vi "FolderMon stop.vi"(4 "error in (no error)":errorcluster) -> (0 "error out":errorcluster)   [LabVIEW 2011]
uses:
  FolderMon events.ctl
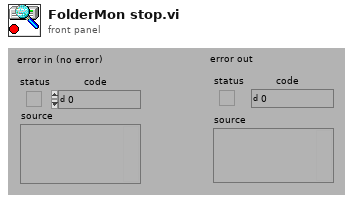
[diagram p1: front panel]
types:
  T1 = typedef "FolderMon events.ctl" = enum16{"stop", "update"}
  T2 = enum32{"Bad", "Idle", "Run top level", "Running"}
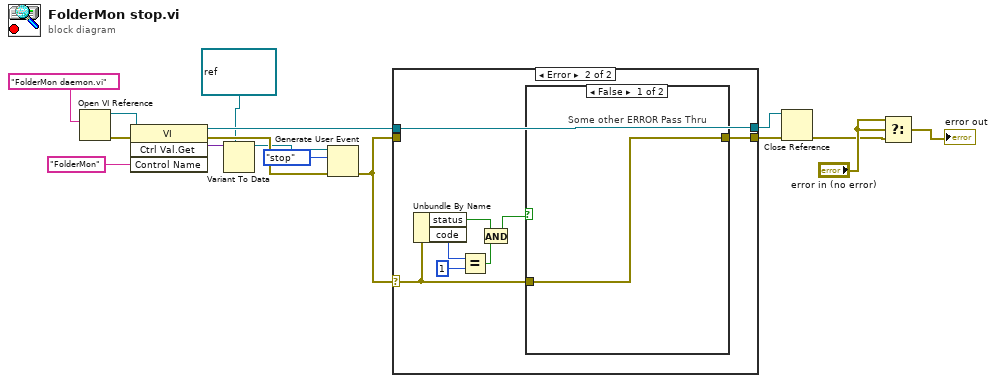
[diagram p0: block diagram]
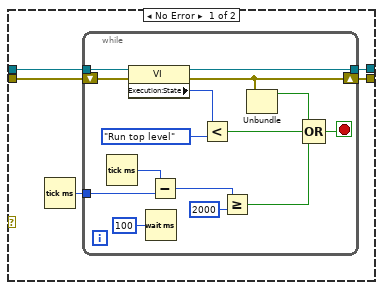
[diagram p2: hidden frame]
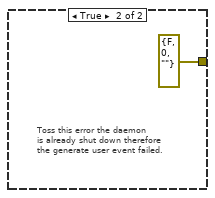
[diagram p3: hidden frame]
diagram:
  w3 = refnum<user-event> refnum items=["stop", "update"] ("FolderMon")
  n1 = Open VI Reference(vi path="FolderMon daemon.vi") -> (vi reference=w15:refnum<vi>, error out=w14:errorcluster)  [unwired: 1 in, 4 out]
  n2 = invoke class="VI" method="Ctrl Val.Get"(reference=w15, error in=w14, "Control Name"="FolderMon") -> (reference out=w12:refnum<vi>, error out=w9:errorcluster, "Get Control Value Variant"=w2:variant)  [unwired: 1 in, 1 out]
  n3 = Variant To Data(type=w3, Variant=w2) -> (data=w1:refnum<user-event>)  [unwired: 1 in, 1 out]
  n4 = Generate User Event(user event=w1, event data cluster=FolderMon_events."stop" ("event data"), error in=w9) -> (error out=w7:errorcluster)  [unwired: 1 out]
  n5 = case shown="Error" w7 {
    selector: w7 -> [_ w38]
    tunnel: w12 -> [w21 w37]
    tunnel: [w19 w39] -> w11
    tunnel: [w18 w37] -> w10
    tunnel: w7 -> [w17 _]
    frame No Error {
      n6 = Tick Count (ms)() -> (millisecond timer value=w20:u32)
      n7 = while {
        shift-right: [w27] -> w19
        shift-left: w17 -> [w33]
        tunnel: w21 -> [w34]
        tunnel: w20 -> [w31]
        tunnel: [w22] -> w18
        stop <- w23 stop-if-true
        n8 = Tick Count (ms)() -> (millisecond timer value=w32:u32)
        n9 = property class="VI"(reference=w34, error in=w33) -> (reference out=w22:refnum<vi>, error out=w27:errorcluster, "Execution:State"=w36:T2)
        n10 = Wait (ms)(milliseconds to wait=u32 100) -> ()  [unwired: 1 out]
        n11 = Subtract(x=w32, y=w31) -> (x-y=w29:u32)
        n12 = Less?(x=w36, y=T2."Run top level") -> (x < y?=w25:bool)
        n13 = Greater Or Equal?(x=w29, y=u32 2000) -> (x >= y?=w24:bool)
        n14 = Unbundle(w27) -> ("status"=w26:bool)  [unwired: 2 out]
        n15 = Compound Arithmetic op=OR(w26, w25, w24) -> (w23:bool)
      }
    }
    frame Error {
      n16 = Unbundle By Name(w38) -> ("status"=w44:bool, "code"=w42:i32)
      n17 = Equal?(x=w42, y=1) -> (x = y?=w41:bool)
      n18 = And(x=w44, y=w41) -> (x .and. y?=w43:bool)
      n19 = case shown="False" w43 {
        tunnel: [w45 errorcluster {"status"=FALSE, "code"=0, "source"=""} ("error IO")] -> w39
        tunnel: w38 -> [w45 _]
        frame False {
          # "Some other ERROR Pass Thru"
        }
        frame True {
          # "Toss this error the daemon\nis already shut down therefore\nthe generate user event failed."
        }
      }
    }
  }
  n20 = Close Reference(reference=w10, error in (no error)=w11) -> (error out=w5:errorcluster)
  n21 = Select(t="error in (no error)", s="error in (no error)", f=w5) -> (s? t:f=→"error out":errorcluster)
